vi "Convert 2D Array to 1D Array.vi"(11 "Array in":dbl[][](array[numeric])) -> (3 "Array out":dbl[](array[numeric]))   [LabVIEW 2021]
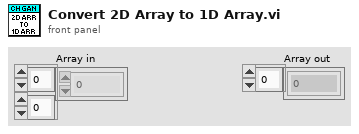
[diagram p1: front panel]
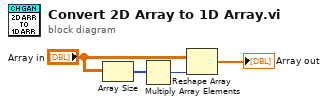
[diagram p0: block diagram]
diagram:
  n1 = Array Size(array="Array in") -> (size(s)=w2:i32[])
  n2 = Multiply Array Elements(1:w2) -> (0:w1:i32)
  n3 = Reshape Array("Array in", w1) -> (→"Array out":dbl[])
